vi "PolishVision.vi"(11 "Refnum in":T1) -> (3 "Refnum out":T1)   [LabVIEW 2015]
uses:
  <vilib>/vision/Image Controls.llb/IMAQ Image.ctl
  <vilib>/vision/NI_Vision_Development_Module.lvlib
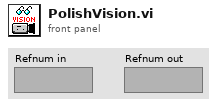
[diagram p1: front panel]
types:
  T1 = typedef "IMAQ Image.ctl" = refnum<image>
  T2 = cluster{"Position":cluster{"X":sgl, "Y":sgl}, "Radius":dbl, "Score":dbl}[]
  T3 = cluster{"Circles[0]":cluster{"Position":cluster{"X":sgl, "Y":sgl}, "Radius":dbl, "Score":dbl}, "Circles[1]":cluster{"Position":cluster{"X":sgl, "Y":sgl}, "Radius":dbl, "Score":dbl}, "Circles[2]":cluster{"Position":cluster{"X":sgl, "Y":sgl}, "Radius":dbl, "Score":dbl}, "Circles[3]":cluster{"Position":cluster{"X":sgl, "Y":sgl}, "Radius":dbl, "Score":dbl}, "Circles[4]":cluster{"Position":cluster{"X":sgl, "Y":sgl}, "Radius":dbl, "Score":dbl}, "Circles[5]":cluster{"Position":cluster{"X":sgl, "Y":sgl}, "Radius":dbl, "Score":dbl}, "Circles[6]":cluster{"Position":cluster{"X":sgl, "Y":sgl}, "Radius":dbl, "Score":dbl}, "Circles[7]":cluster{"Position":cluster{"X":sgl, "Y":sgl}, "Radius":dbl, "Score":dbl}, "Circles[8]":cluster{"Position":cluster{"X":sgl, "Y":sgl}, "Radius":dbl, "Score":dbl}}
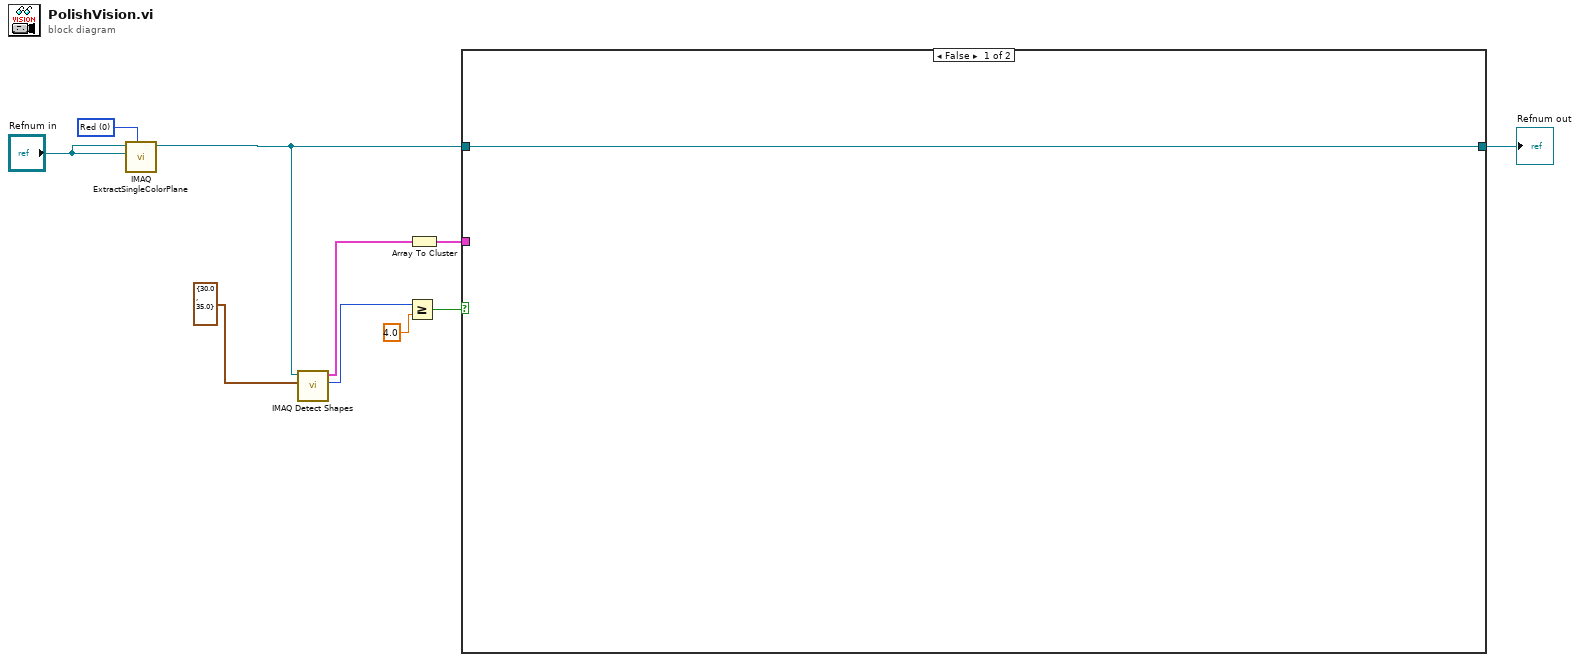
[diagram p0: block diagram]
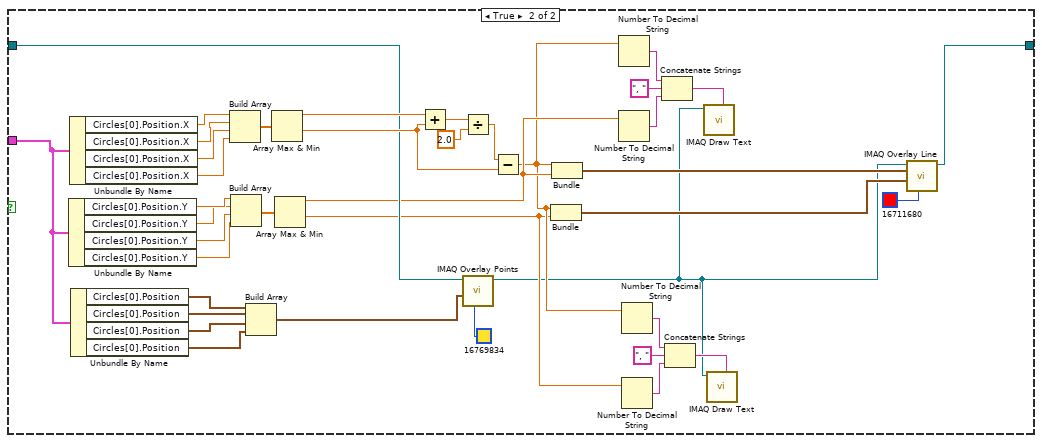
[diagram p2: hidden frame]
diagram:
  w10 = 0 items=["Red", "Green", "Blue", "Hue", "Saturation", "Luminance", "Value", "Intensity"] ("Color Plane")
  n1 = call "IMAQ ExtractSingleColorPlane"("Color Plane"=w10, "Image Dst"="Refnum in", "Image Src"="Refnum in") -> ("Image Dst Out"=w4:T1)  [unwired: 7 in, 1 out]
  n2 = call-poly "IMAQ Detect Shapes"("Circle Descriptor"=cluster{"Min Radius":dbl, "Max Radius":dbl} {"Min Radius"=30.0, "Max Radius"=35.0}, "Image"=w4) -> ("Number of Matches Returned"=w1:i32, "Circles"=w2:T2)  [unwired: 7 in, 1 out]
  n3 = Greater Or Equal?(x=w1, y=4.0) -> (x >= y?=w7:bool)
  n4 = Array To Cluster(array=w2) -> (cluster=w5:T3)
  n5 = case shown="False" w7 {
    tunnel: w4 -> [w11 w24]
    tunnel: [w11 w42] -> w6
    tunnel: w5 -> [_ w30]
    frame False {
    }
    frame True {
      n6 = Unbundle By Name(w30) -> ("Circles[0].Position.Y"=w29:sgl, "Circles[0].Position.Y"=w28:sgl, "Circles[0].Position.Y"=w27:sgl, "Circles[0].Position.Y"=w26:sgl)
      n7 = Unbundle By Name(w30) -> ("Circles[0].Position.X"=w34:sgl, "Circles[0].Position.X"=w33:sgl, "Circles[0].Position.X"=w32:sgl, "Circles[0].Position.X"=w31:sgl)
      n8 = Unbundle By Name(w30) -> ("Circles[0].Position"=w40:cluster{"X":sgl, "Y":sgl}, "Circles[0].Position"=w39:cluster{"X":sgl, "Y":sgl}, "Circles[0].Position"=w38:cluster{"X":sgl, "Y":sgl}, "Circles[0].Position"=w37:cluster{"X":sgl, "Y":sgl})
      n9 = Build Array(w34, w33, w32, w31) -> (w50:sgl[])
      n10 = Build Array(w29, w28, w27, w26) -> (w49:sgl[])
      n11 = Build Array(w40, w39, w38, w37) -> (w36:cluster{"X":sgl, "Y":sgl}[])
      n12 = Array Max & Min(array=w50) -> (max value=w48:sgl, min value=w44:sgl)  [unwired: 2 out]
      n13 = Array Max & Min(array=w49) -> (max value=w23:sgl, min value=w13:sgl)  [unwired: 2 out]
      n14 = Add(x=w48, y=w44) -> (x+y=w47:sgl)
      n15 = Divide(x=w47, y=sgl 2.0) -> (x/y=w45:sgl)
      n16 = call "IMAQ Overlay Points"("Color"=u32 16769834, "Array of Points"=w36, "Image"=w24) -> ("Image Out"=w12:T1)  [unwired: 7 in, 1 out]
      n17 = Subtract(x=w45, y=w44) -> (x-y=w14:sgl)
      n18 = Bundle(w14, w13) -> (w43:cluster{sgl, sgl})  [unwired: 1 in]
      n19 = Bundle(w14, w23) -> (w25:cluster{sgl, sgl})  [unwired: 1 in]
      n20 = Number To Decimal String(number=w14) -> (decimal integer string=w22:string)  [unwired: 1 in]
      n21 = Number To Decimal String(number=w23) -> (decimal integer string=w21:string)  [unwired: 1 in]
      n22 = Number To Decimal String(number=w14) -> (decimal integer string=w15:string)  [unwired: 1 in]
      n23 = Number To Decimal String(number=w13) -> (decimal integer string=w16:string)  [unwired: 1 in]
      n24 = Concatenate Strings(w22, ", " ("string"), w21) -> (w19:string)
      n25 = Concatenate Strings(w15, ", " ("string"), w16) -> (w18:string)
      n26 = call "IMAQ Draw Text"("String"=w19, "Image Src"=w12) -> ()  [unwired: 6 in, 4 out]
      n27 = call "IMAQ Draw Text"("String"=w18, "Image Src"=w12) -> ()  [unwired: 6 in, 4 out]
      n28 = call "IMAQ Overlay Line"("Color"=u32 16711680, "End Point"=w43, "Start Point"=w25, "Image"=w12) -> ("Image Out"=w42:T1)  [unwired: 6 in, 1 out]
    }
  }
  "Refnum out" <- w6
